vi "array-indexing.vi"() -> ()   [LabVIEW 2020]
panel:
  in  "index":i32=2
  out "element 5":u8
  out "element 4":u8
  out "element 3":u8
  out "element 2":u8
  out "element1":u8
  in  "Data":u8[](array[numeric])
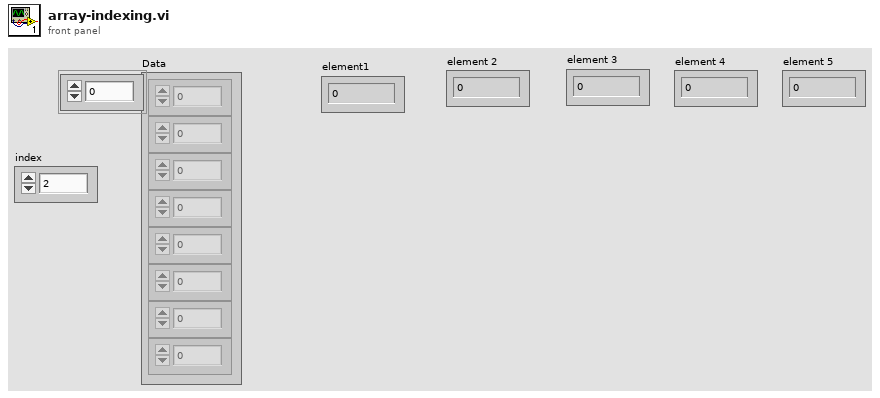
[diagram p1: front panel]
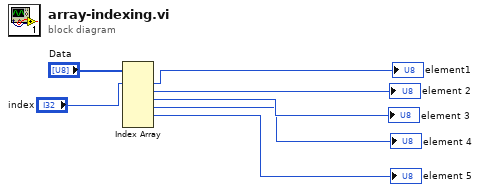
[diagram p0: block diagram]
diagram:
  n1 = Index Array(array="Data", index #1="index") -> (element #1=→"element1":u8, element #2=→"element 2":u8, element #3=→"element 3":u8, element #4=→"element 4":u8, element #5=→"element 5":u8)  [unwired: 5 in, 1 out]
